vi "01 - Custom Debugging.vi"   [LabVIEW 2021]
panel:
  # "Open Block Diagram to Debug Code\nCtl + E (instructions on diagram)"
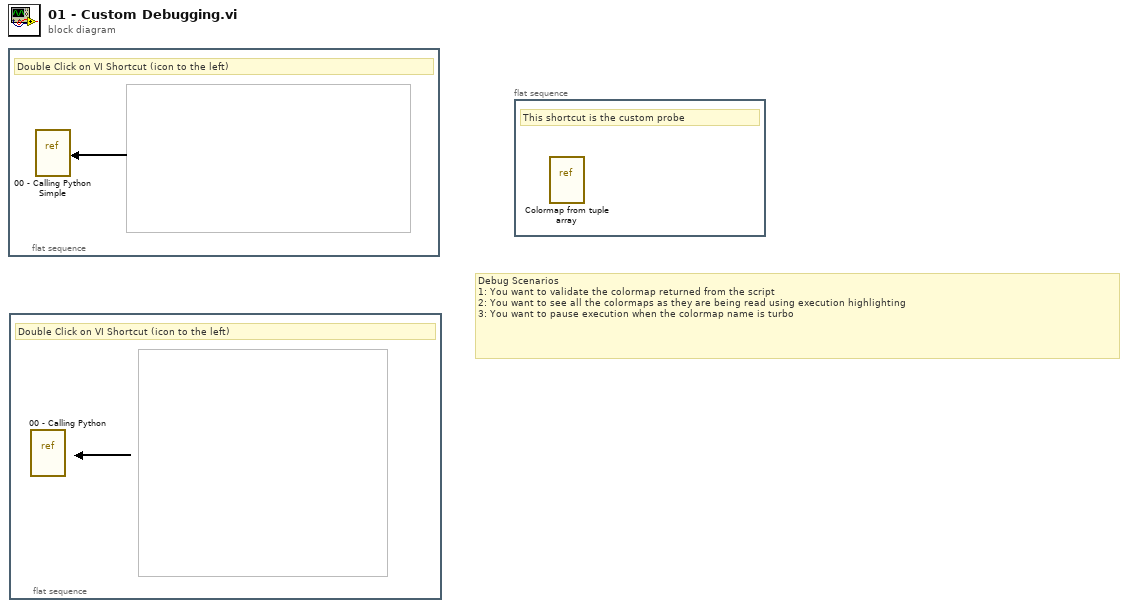
[diagram p0: block diagram]
diagram:
  # "Debug Scenarios\n1: You want to validate the colormap returned from the script\n2: You want to see all the colormaps as they are being read using execution highlighting\n3: You want to pause execution when the colormap name is turbo"
  n1 = flat-sequence {
    frame #0 {
      # "Double Click on VI Shortcut (icon to the left)"
      n2 = vi-ref "00 - Calling Python Simple.vi"() -> ()  [unwired: 1 out]
    }
  }
  n3 = flat-sequence {
    frame #0 {
      # "Double Click on VI Shortcut (icon to the left)"
      n4 = vi-ref "00 - Calling Python.vi"() -> ()  [unwired: 1 out]
    }
  }
  n5 = flat-sequence {
    frame #0 {
      # "This shortcut is the custom probe"
      n6 = vi-ref "Colormap from tuple array.vi"() -> ()  [unwired: 1 out]
    }
  }
